vi "Read B-Scan Info Array.vi"(8 "error in (no error)":errorcluster, 11 "Read in":refnum<class "Read.lvclass">) -> (0 "error out":errorcluster, 2 "B-Scan Info Array":T1[](array[typedef]), 3 "Read out":refnum<class "Read.lvclass">)   [LabVIEW 2014, in "Read.lvclass"]
uses:
  Read.lvclass
  BScan.ctl
  Read.lvclass/Read.ctl
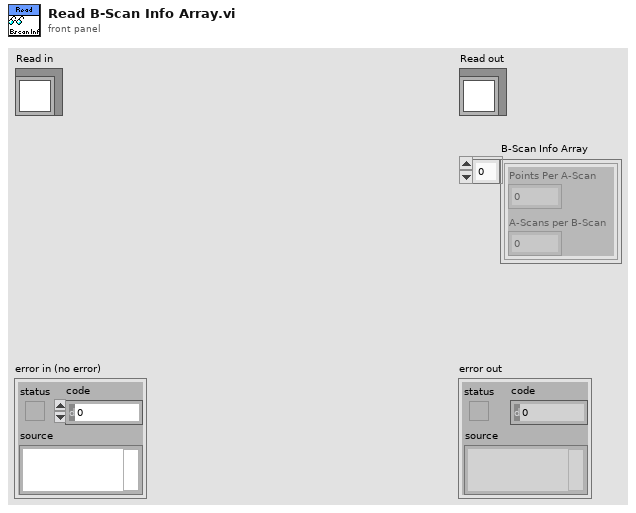
[diagram p1: front panel]
types:
  T1 = typedef "Read.lvclass/BScan.ctl" = cluster{"Points Per A-Scan":dbl, "A-Scans per B-Scan":dbl}
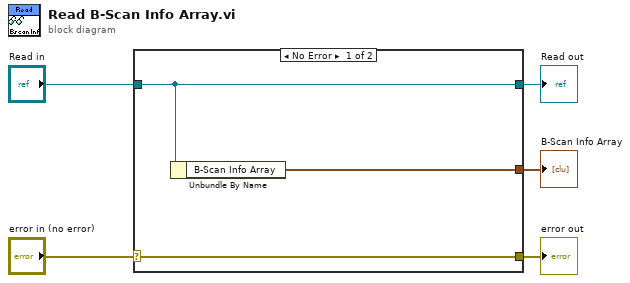
[diagram p0: block diagram]
diagram:
  n1 = case shown="No Error" "error in (no error)" {
    selector: "error in (no error)" -> [w8 w9]
    tunnel: [w8 w9] -> w4
    tunnel: [w7 w10] -> w2
    tunnel: "Read in" -> [w7 w10]
    tunnel: [w6 _] -> w1
    frame No Error {
      n2 = Unbundle By Name(w7) -> ("B-Scan Info Array"=w6:T1[])
    }
    frame Error {
    }
  }
  "error out" <- w4
  "Read out" <- w2
  "B-Scan Info Array" <- w1
